vi "Tree_IndentItem.vi"(8 "Error In":errorcluster, 10 "TagToIndent":string, 11 "Tree Refnum":refnum<vi>) -> (0 "Error Out":errorcluster, 3 "Tree Refnum OUT":refnum<vi>)   [LabVIEW 2012]
doc: "SciScan 1.2 160622"
panel:
  in  "Tree":string(tree)
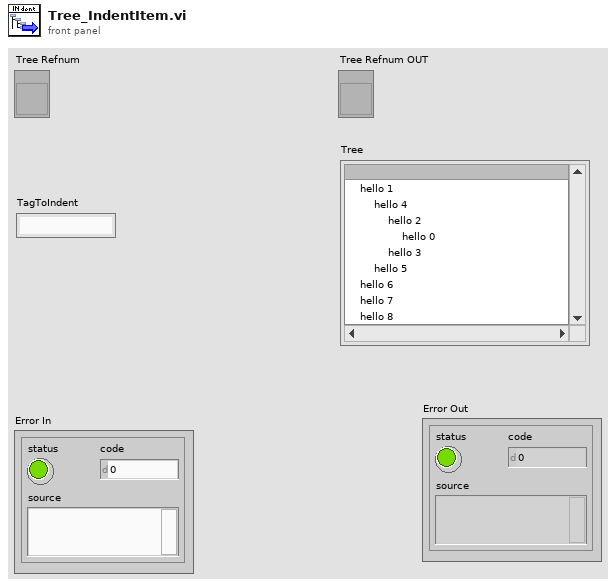
[diagram p1: front panel]
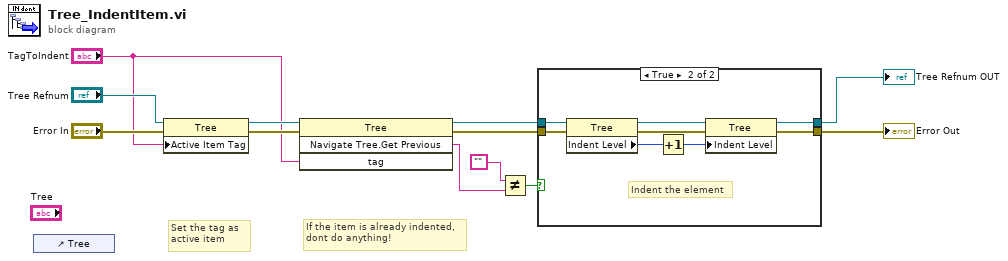
[diagram p0: block diagram]
diagram:
  # "If the item is already indented,\ndont do anything!"
  # "Set the tag as active item"
  n1 = control-ref of="Tree"() -> ()  [unwired: 1 out]
  n2 = property class="Tree"(reference="Tree Refnum", error in="Error In", "Active Item Tag"="TagToIndent") -> (reference out=w3:refnum<vi>, error out=w4:errorcluster)
  n3 = invoke class="Tree" method="Navigate Tree.Get Previous"(reference=w3, error in=w4, "tag"="TagToIndent") -> (reference out=w5:refnum<vi>, error out=w6:errorcluster, "Navigate Tree:Get Previous"=w9:string)  [unwired: 1 in, 1 out]
  n4 = Not Equal?(x="", y=w9) -> (x != y?=w8:bool)
  n5 = case shown="True" w8 {
    tunnel: [w14 w22] -> w12
    tunnel: [w13 w21] -> w11
    tunnel: w6 -> [w13 w16]
    tunnel: w5 -> [w14 w15]
    frame False {
    }
    frame True {
      # "Indent the element"
      n6 = property class="Tree"(reference=w15, error in=w16) -> (reference out=w17:refnum<vi>, error out=w20:errorcluster, "Indent Level"=w19:i32)
      n7 = Increment(x=w19) -> (x+1=w18:i32)
      n8 = property class="Tree"(reference=w17, error in=w20, "Indent Level"=w18) -> (reference out=w22:refnum<vi>, error out=w21:errorcluster)
    }
  }
  "Error Out" <- w11
  "Tree Refnum OUT" <- w12
